vi "PRESSdll.vi"(8 "error in (no error)":errorcluster, 9 "z":dbl[](array[numeric]), 10 "D":dbl, 11 "t":dbl) -> (0 "error out":errorcluster, 3 "p out":dbl)   [LabVIEW 2021]
doc: "subroutine PRESSdll(t, D, z, p)\n\nCompute pressure as a function of temperature, density, and composition. See warning in suroutines THERM or ALLPROPS.\n\nINPUTS:\nt -- Temperature [K]\nD -- Molar density [mol/L]\nz -- Composition (array of mole fractions)\n\nOUTPUTS:\np -- Pressure [kPa]"
uses:
  REFPROP.dll
panel:
  # "REFPROP-PRESSdll.vi"
  # "void  PRESSdll(double *t, double *D, double *z, double *p)"
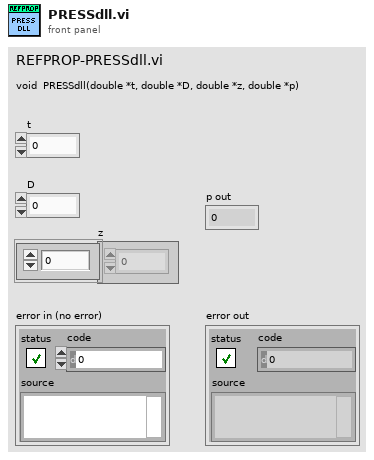
[diagram p1: front panel]
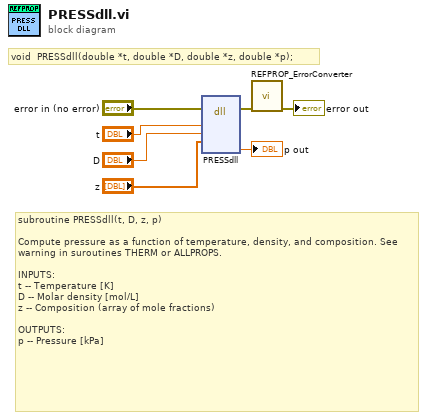
[diagram p0: block diagram]
diagram:
  # "void  PRESSdll(double *t, double *D, double *z, double *p);"
  # "subroutine PRESSdll(t, D, z, p)\n\nCompute pressure as a function of temperature, density, and composition. See warning in suroutines THERM or ALLPROPS.\n\nINPUTS:\nt -- Temperature [K]\nD -- Molar density [mol/L]\nz -- Composition (array of mole fractions)\n\nOUTPUTS:\np -- Pressure [kPa]"
  n1 = dll-call lib="C:/Users/lauria/OneDrive - National Institute of Standards and Technology (NIST)/LabVIEW Projects/7 REFPROP/REFPROP-wrappers-master/REFPROP-wrappers-master/wrappers/Labview/REFPROP/REFPROP.*" fn="PRESSdll"(error in="error in (no error)", "t"="t", "D"="D", "z"="z") -> (error out=w3:errorcluster, "p"=→"p out":dbl)  [unwired: 7 in, 1 out]
  n2 = call "REFPROP_ErrorConverter.vi"("error in (no error)"=w3) -> ("error out"=→"error out":errorcluster)  [unwired: 10 in]
